vi "txtFile to Excel.vi"(10 "ResultArrayIn":string[](array[string])) -> ()   [LabVIEW 2017]
uses:
  <vilib>/Utility/NIReport.llb/NI_report.lvclass
  <vilib>/addons/_office/NI_ReportGenerationToolkit.lvlib
  <vilib>/Utility/NIReport.llb/Excel/NI_Excel.lvclass
  <vilib>/addons/_office/excel.llb/Excel Get Data (str).vi
  <vilib>/addons/_office/excel.llb/Excel Easy Table (str).vi
panel:
  in  "Table":string[][](table)=[["1", "2", "3", "4", "5", "6", "7", "8", "9", "10"], ["10", "11", "12", "13", "14", "15", "16", "17", "18", "19"], ["20", "21", "22", "23", "24", "25", "26", "27", "28", "29"], ["30", "31", "32", "33", "34", "35", "36", "37", "38", "39"]]
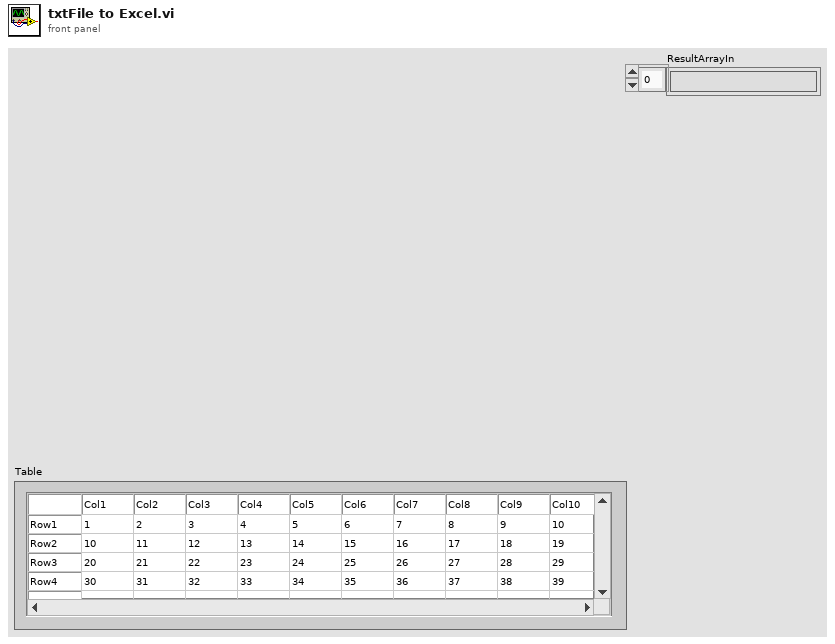
[diagram p1: front panel]
types:
  T1 = enum16{"Standard Report", "HTML", "Word", "Excel"}
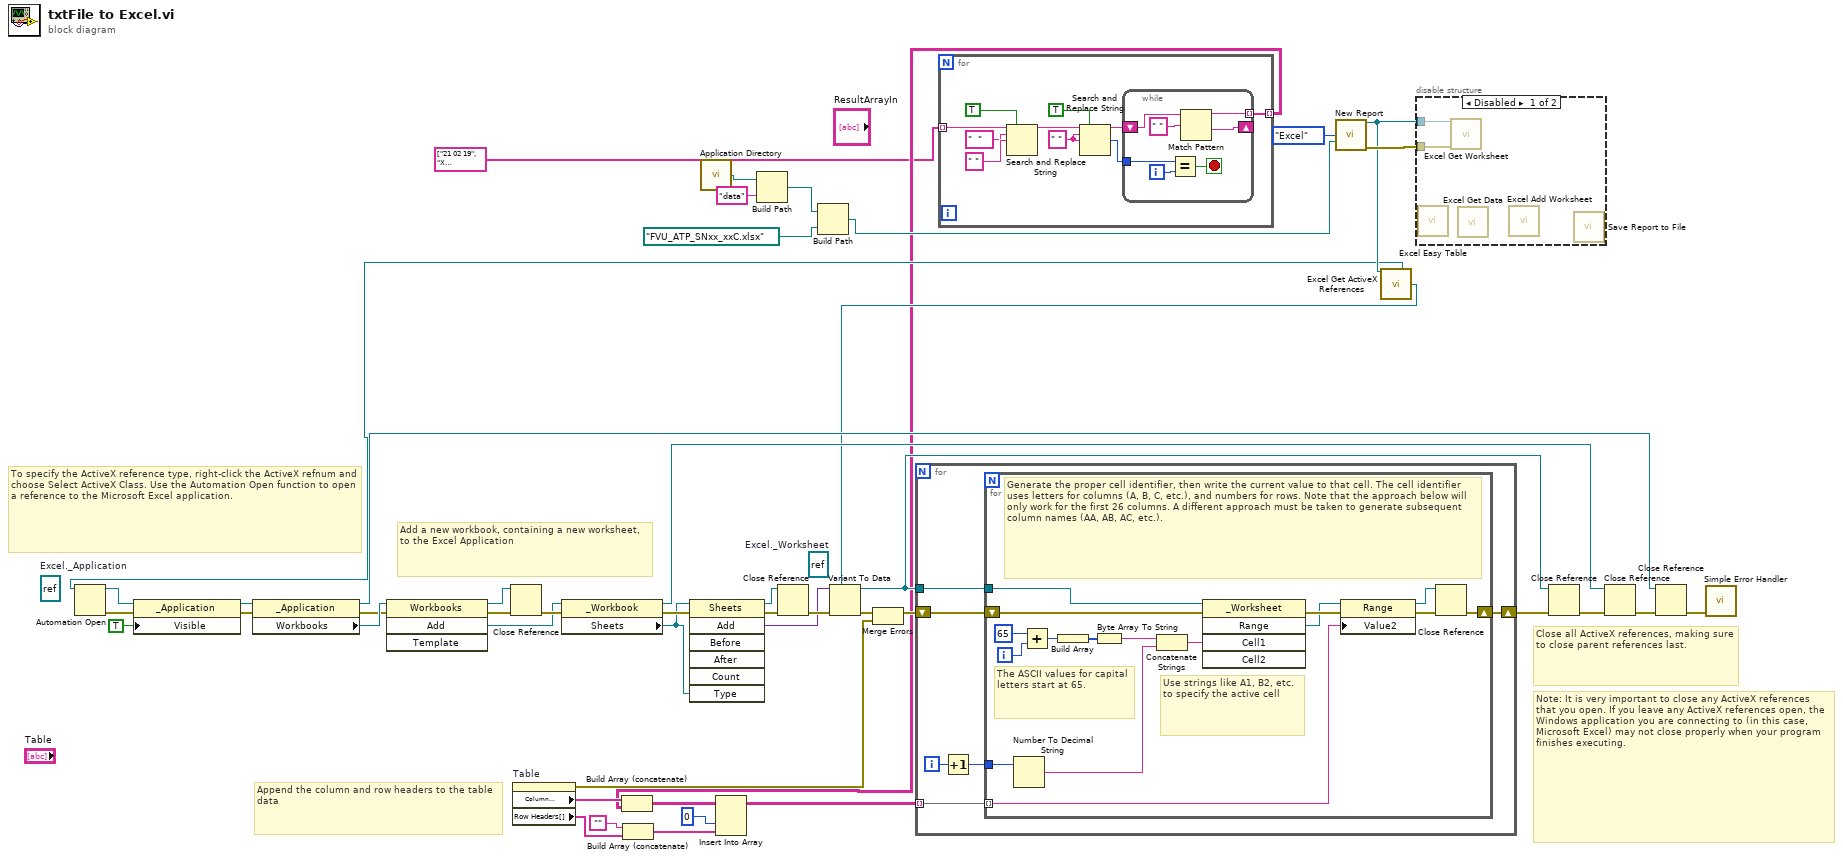
[diagram p0: block diagram]
diagram:
  (unwired) refnum<k7> refnum  # Excel._Worksheet
  (unwired) refnum<k7> refnum  # Excel._Application
  # "Note: It is very important to close any ActiveX references that you open. If you leave any ActiveX references open, the Windows application you are connecting to (in this case, Microsoft Excel) may not close properly when your program finishes executing."
  # "Add a new workbook, containing a new worksheet, to the Excel Application"
  # "Append the column and row headers to the table data"
  # "Close all ActiveX references, making sure to close parent references last."
  # "To specify the ActiveX reference type, right-click the ActiveX refnum and choose Select ActiveX Class. Use the Automation Open function to open a reference to the Microsoft Excel application."
  n1 = property on="Table" class="Tbl (strict)"() -> (error out=w9:errorcluster, "Column Headers[]"=w14:string[], "Row Headers[]"=w8:string[])  [unwired: 2 in, 1 out]
  n2 = Build Array (concatenate)("", w8) -> (w7:string[])
  n3 = call <vilib>:"Application Directory.vi"() -> ("Application Directory"=w45:path)
  n4 = Build Path(base path=w45, name or relative path="data") -> (appended path=w42:path)
  n5 = Build Path(base path=w42, name or relative path=path "FVU_ATP_SNxx_xxC.xlsx") -> (appended path=w41:path)
  n6 = for {
    tunnel: string[] ["21 02 19", "X 41.000000", "Mag FB  ADCReset  ADCSet", "1.012081 630 2993 2261 3552 876 1662 2037 ", "0.910265 647 2980 2281 3531 867 1672 2039 ", "0.809526 662 2964 2302 3506 857 1679 2038 ", "21 02 19", "X 41.000000", "Mag FB  ADCReset  ADCSet", "21 02 19", "X 40.750000", "Mag FB  ADCReset  ADCSet", "21 02 19", "X 41.000000", "Mag FB  ADCReset  ADCSet", "0.707733 680 2954 2331 3498 860 1704 2039 ", "0.606404 694 2937 2355 3471 855 1708 2039 ", "0.505167 709 2920 2376 3450 843 1721 2037 ", "0.403641 732 2911 2393 3427 826 1732 2038 ", "0.302855 741 2895 2411 3404 814 1740 2036 ", "11:20:29  300.000000 0.941008 0.094913 -0.146794 0.695456 -0.319529 -0.316111 -9.303915 -9.303980 -9.305329 14338 ", "0.201144 761 2878 2427 3382 807 1753 2035 ", "11:20:31  200.000000 0.955840 0.114689 -0.156682 0.680074 -0.304788 -0.320841 -9.303915 -9.303980 -9.305329 14338 ", "0.099722 779 2866 2459 3369 805 1768 2038 ", "11:20:33  100.000000 0.958281 0.114689 -0.139409 0.669820 -0.291940 -0.325541 -9.303915 -9.303980 -9.305329 14338 ", "-0.001689 797 2851 2472 3354 796 1782 2039 ", "11:20:35  0.000000 0.973113 0.117130 -0.154241 0.657033 -0.277200 -0.328898 -9.303915 -9.303980 -9.305329 14338 ", "-0.103505 805 2836 2493 3322 773 1784 2038 ", "11:20:37  -100.000000 0.955840 0.117130 -0.151738 0.644856 -0.270760 -0.339671 -9.303915 -9.303980 -9.305329 14338 ", "-0.204279 815 2813 2518 3309 761 1801 2035 ", "11:20:38  -200.000000 0.960784 0.119572 -0.156682 0.634602 -0.257302 -0.347728 -9.303915 -9.303980 -9.305329 14338 ", "-0.306025 832 2798 2534 3295 747 1814 2038 ", "11:20:40  -300.000000 0.941008 0.087527 -0.151738 0.626301 -0.243812 -0.354442 -9.303915 -9.303980 -9.305329 14338 ", "-0.407482 850 2779 2538 3273 721 1818 2037 ", "-0.508510 871 2759 2565 3250 715 1829 2033 ", "-0.610071 881 2749 2577 3237 700 1843 2038 ", "21 02 19", "X 41.000000", "Mag FB  ADCReset  ADCSet", "21 02 19", "X 41.000000", "Mag FB  ADCReset  ADCSet", "21 02 19", "X 41.000000", "Mag FB  ADCReset  ADCSet", "-0.710590 895 2730 2591 3220 676 1860 2038 ", "-0.812395 912 2716 2614 3203 668 1871 2038 ", "-0.913747 929 2700 2633 3186 657 1881 2039 ", "-1.015297 947 2678 2652 3186 658 1908 2039 "] ("Array") -> [w50] mode=indexing
    tunnel: [w53] -> w2 mode=indexing
    w54 = " " ("regular expression")
    n7 = Search and Replace String(replace all?=TRUE ("replace all? (F)"), input string=w50, search string="  " ("regular expression"), replace string=" " ("regular expression")) -> (result string=w49:string)  [unwired: 4 in, 3 out]
    n8 = Search and Replace String(replace all?=TRUE ("replace all? (F)"), input string=w49, search string=w54, replace string=w54) -> (result string=w47:string, number of replacements=w55:i32)  [unwired: 4 in, 2 out]
    n9 = while {
      shift-right: [w61] -> _
      shift-left: w47 -> [w63]
      tunnel: [w60] -> w53 mode=indexing
      tunnel: w55 -> [w59]
      i -> [w57]
      stop <- w58 stop-if-true
      n10 = Equal?(x=w59, y=w57) -> (x = y?=w58:bool)
      n11 = Match Pattern(string=w63, regular expression=" ") -> (before substring=w60:string, after substring=w61:string)  [unwired: 1 in, 2 out]
    }
  }
  n12 = Build Array (concatenate)(w14, w2) -> (w13:string[][])
  n13 = Insert Into Array(array=w13, index (col)=0 ("disabled index (col)"), new element=w7) -> (w11:string[][])  [unwired: 1 in]
  n14 = call <vilib>:"New Report.vi"("report type"=T1."Excel", "template (empty)"=w41) -> ("report out"=w39:refnum<class "NI_report.lvclass">, "error out"=w40:errorcluster)  [unwired: 12 in]
  n15 = call <vilib>:"Excel Get ActiveX References.vi"("report in"=w39) -> ("Excel._Application"=w5:refnum<k7>, "Excel._Worksheet"=w4:refnum<k7>)  [unwired: 8 in, 5 out]
  n16 = Automation Open(Automation Refnum=w5) -> (Automation Refnum=w33:refnum<k7>, error out=w34:errorcluster)  [unwired: 1 in, 2 out]
  n17 = property class="_Application"(reference=w33, error in=w34, "Visible"=TRUE) -> (reference out=w26:refnum<k7>, error out=w28:errorcluster)
  n18 = property class="_Application"(reference=w26, error in=w28) -> (reference out=w23:refnum<k7>, error out=w31:errorcluster, "Workbooks"=w32:refnum<k7>)
  n19 = invoke class="Workbooks" method="Add"(reference=w32, error in=w31) -> (reference out=w29:refnum<k7>, error out=w30:errorcluster, "Add"=w24:refnum<k7>)  [unwired: 2 in, 1 out]
  n20 = Close Reference(reference=w29, error in (no error)=w30) -> (error out=w25:errorcluster)
  n21 = property class="_Workbook"(reference=w24, error in=w25) -> (reference out=w21:refnum<k7>, error out=w16:errorcluster, "Sheets"=w3:refnum<k7>)
  n22 = invoke class="Sheets" method="Add"(reference=w3, error in=w16, "Type"=w3) -> (reference out=w18:refnum<k7>, error out=w19:errorcluster, "Add"=w17:variant)  [unwired: 4 in, 4 out]
  n23 = Close Reference(reference=w18, error in (no error)=w19) -> (error out=w20:errorcluster)
  n24 = Variant To Data(error in=w20, type=w4, Variant=w17) -> (data=w22:refnum<k7>, error out=w15:errorcluster)
  n25 = Merge Errors(w15, w9) -> (w10:errorcluster)
  n26 = for {
    shift-right: [w68] -> w35
    shift-left: w10 -> [w69]
    tunnel: w22 -> [w67]
    tunnel: w11 -> [w64] mode=indexing
    i -> [w66]
    n27 = Increment(x=w66) -> (x+1=w65:i32)
    n28 = for {
      shift-right: [w81] -> w68
      shift-left: w69 -> [w79]
      tunnel: w67 -> [w78]
      tunnel: w65 -> [w73]
      tunnel: w64 -> [w83] mode=indexing
      i -> [w74]
      # "Use strings like A1, B2, etc. to specify the active cell"
      # "The ASCII values for capital letters start at 65."
      # "Generate the proper cell identifier, then write the current value to that cell. The cell identifier uses letters for columns (A, B, C, etc.), and numbers for rows. Note that the approach below will only work for the first 26 columns. A different approach must be taken to generate subsequent column names (AA, AB, AC, etc.)."
      n29 = Number To Decimal String(number=w73) -> (decimal integer string=w71:string)  [unwired: 1 in]
      n30 = Add(x=65, y=w74) -> (x+y=w76:i32)
      n31 = Build Array(w76) -> (w75:i32[])
      n32 = Byte Array To String(unsigned byte array=w75) -> (string=w72:string)
      n33 = Concatenate Strings(w72, w71) -> (w70:string)
      n34 = invoke class="_Worksheet" method="Range"(reference=w78, error in=w79, "Cell1"=w70) -> (error out=w85:errorcluster, "Range"=w84:refnum<k7>)  [unwired: 2 in, 3 out]
      n35 = property class="Range"(reference=w84, error in=w85, "Value2"=w83) -> (reference out=w80:refnum<k7>, error out=w82:errorcluster)
      n36 = Close Reference(reference=w80, error in (no error)=w82) -> (error out=w81:errorcluster)
    }
  }
  n37 = disable-structure shown="Disabled" {
    disable-tunnel: w40 -> [w87 _]
    disable-tunnel: w39 -> [w86 _]
    frame Disabled {
      n38 = call-poly <vilib>:"Excel Easy Table.vi"() -> ()  [unwired: 11 in, 5 out]
      n39 = call <vilib>:"Excel Get Worksheet.vi"("report in"=w86, "error in (no error)"=w87) -> ()  [unwired: 12 in, 2 out]
      n40 = call-poly <vilib>:"Excel Get Data.vi"() -> ()  [unwired: 13 in, 3 out]
      n41 = call <vilib>:"Excel Add Worksheet.vi"() -> ()  [unwired: 14 in, 2 out]
      n42 = call-dynamic "Save Report to File.vi"() -> ()  [unwired: 14 in, 2 out]
    }
    frame Enabled {
    }
  }
  n43 = Close Reference(reference=w22, error in (no error)=w35) -> (error out=w38:errorcluster)
  n44 = Close Reference(reference=w21, error in (no error)=w38) -> (error out=w37:errorcluster)
  n45 = Close Reference(reference=w23, error in (no error)=w37) -> (error out=w36:errorcluster)
  n46 = call <vilib>:"Simple Error Handler.vi"("error in (no error)"=w36) -> ()  [unwired: 4 in, 5 out]
